vi "_Write XML Table.vi"(4 "error in":errorcluster, 6 "Table Type":u8, 7 "Table (2D-DBL)":dbl[][](array[numeric])) -> (0 "error out":errorcluster, 3 "XML String":string)   [LabVIEW 2015]
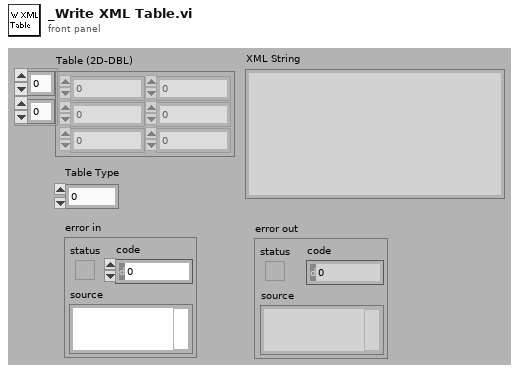
[diagram p1: front panel]
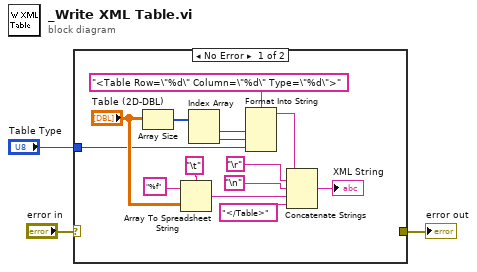
[diagram p0: block diagram]
diagram:
  n1 = case shown="No Error" "error in" {
    selector: "error in" -> [_ w18]
    tunnel: [_ w18] -> w2
    tunnel: "Table Type" -> [w6 _]
    frame No Error {
      n2 = Array Size(array="Table (2D-DBL)") -> (size(s)=w17:i32[])
      n3 = Array To Spreadsheet String(delimiter (Tab)="\t", array="Table (2D-DBL)", 3:"%f" ("format string")) -> (spreadsheet string=w8:string)
      n4 = Index Array(array=w17) -> (element #1=w16:i32, element #2=w15:i32)  [unwired: 2 in]
      n5 = Format Into String(format string="<Table Row=\"%d\" Column=\"%d\" Type=\"%d\">", w16, w15, w6) -> (resulting string=w13:string)  [unwired: 2 in, 1 out]
      n6 = Concatenate Strings(w13, "\r", "\n", w8, "</Table>" ("format string")) -> (→"XML String":string)
    }
    frame Error {
    }
  }
  "error out" <- w2
